vi "Read cfg cluster.vi"(8 "error in (no error)":errorcluster, 11 "Get Serialized Device Configuration MSG in":refnum<class "Get Serialized Device Configuration MSG.lvclass">) -> (0 "error out":errorcluster, 2 "cluster":T1={"ID"="", "type"="", "label"="", "SN"="", "controller_"=FALSE, "Addr"="", "Model"="", "Device Active"=TRUE}, 3 "Get Serialized Device Configuration MSG out":refnum<class "Get Serialized Device Configuration MSG.lvclass">)   [LabVIEW 2015, in "DAQ Device.lvlib" / "Get Serialized Device Configuration MSG.lvclass"]
uses:
  Get Serialized Device Configuration MSG.lvclass
  DAQ Device/Cfg Msg.ctl
  Get Serialized Device Configuration MSG.lvclass/Get Serialized Device Configuration MSG.ctl
  DAQ Device.lvlib
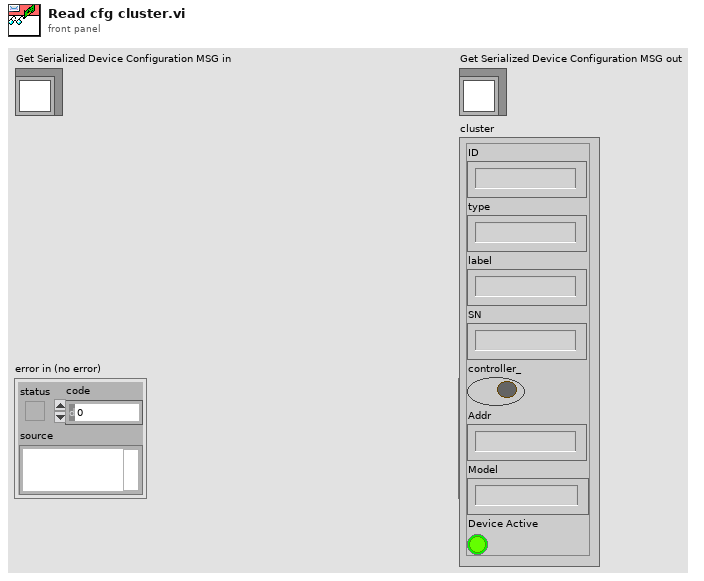
[diagram p1: front panel]
types:
  T1 = typedef "DAQ Device.lvlib/Cfg Msg.ctl" = cluster{"ID":string, "type":string, "label":string, "SN":string, "controller_":bool, "Addr":string, "Model":string, "Device Active":bool}
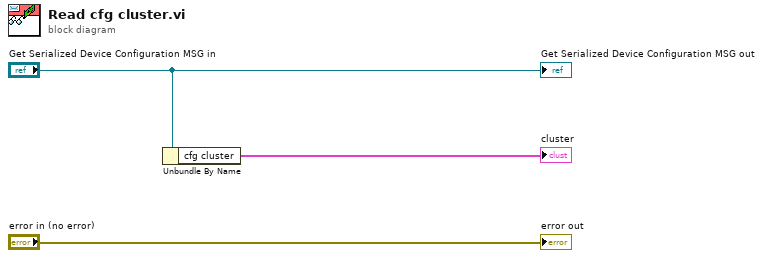
[diagram p0: block diagram]
diagram:
  n1 = Unbundle By Name("Get Serialized Device Configuration MSG in") -> ("cfg cluster"=→"cluster":T1)
  "error out" <- "error in (no error)"
  "Get Serialized Device Configuration MSG out" <- "Get Serialized Device Configuration MSG in"
